vi "move variable to one side.vi"(1 "i to ii ? (ii to i)":bool, 2 "index":i8, 3 "system of equation":T1) -> (0 "system of equation":T1)   [LabVIEW 2009]
uses:
  polynomial equation.ctl
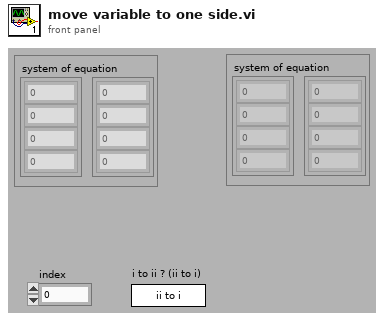
[diagram p1: front panel]
types:
  T1 = typedef "polynomial equation.ctl" = cluster{"i":dbl[], "ii":dbl[]}
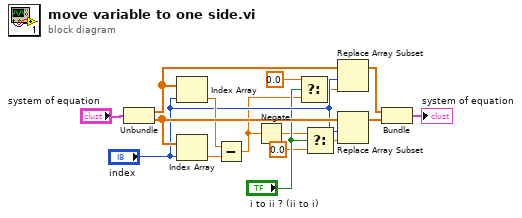
[diagram p0: block diagram]
diagram:
  n1 = Unbundle("system of equation") -> ("i"=w13:dbl[], "ii"=w12:dbl[])
  n2 = Index Array(array=w13, index="index") -> (element=w10:dbl)
  n3 = Index Array(array=w12, index="index") -> (element=w11:dbl)
  n4 = Subtract(x=w10, y=w11) -> (x-y=w1:dbl)
  n5 = Negate(x=w1) -> (-x=w2:dbl)
  n6 = Select(t=0.0, s="i to ii ? (ii to i)", f=w1) -> (s? t:f=w7:dbl)
  n7 = Select(t=w2, s="i to ii ? (ii to i)", f=0.0) -> (s? t:f=w6:dbl)
  n8 = Replace Array Subset(array=w13, new element=w7, index="index") -> (w14:dbl[])
  n9 = Replace Array Subset(array=w12, new element=w6, index="index") -> (w15:dbl[])
  n10 = Bundle("i"=w14, "ii"=w15) -> (→"system of equation":cluster{"i":dbl[], "ii":dbl[]})  [unwired: 1 in]
